vi "ArmController.vi"(7 "Disabled":bool, 9 "Robot Mode":T1, 10 "SensorInputData":T6, 11 "HMI to Control":T2={"RightDriveValue"=0.0, "LeftDriveValue"=0.0, "Arm Manual "=0.0, "Stacker Manual "=0.0, "Claw Manual "=0.0, "ClawSlightOpenNumber"=0, "Intake Value "=0.0, "Arm States"=enum."4 Tote", "Claw States"=enum."Claw Manual ", "Intake Man. or Sense"=enum."Sensing", "Stacker in Manual?"=FALSE, "Drop Stack? "=FALSE, "Tusk Up Request"=FALSE, "Tusk Down Request"=FALSE, "Inver. Wheels  In Request"=FALSE, "Inverse. Wheels Out Request "=FALSE, "Get Out of Manual Control"=FALSE, "Exit Score State"=FALSE, "DriveStraight Help?"=FALSE, "Stacker Shut Off No."=0, "Stacker Need Off?"=FALSE, "Collecting?"=FALSE, "Go to Hover"=FALSE, "Stack Clamp Lock "=FALSE, "Stack Clamp Unlock "=FALSE, "Claw Intake Value "=0.0, "Stack Clamp Lock No. "=0, "Steal Can (ruin their day?)"=FALSE, "Retract (have mercy?)"=FALSE, "Can Grab No. "=0, "Wench Value to Control "=0.0}) -> (2 "Device has arrived":bool, 3 "Final Arm Output":dbl)   [LabVIEW 2014]
uses:
  Typedefs/SensorInputData.ctl
  Typedefs/HMI_to_Control.ctl
  Typedefs/Arm States.ctl
  Typedefs/ClawStates.ctl
  Typedefs/IntakeWheelSenseOrManual.ctl
  <vilib>/Rock Robotics/WPI/DriverStation/WPI_DriverStationRobotMode2.ctl
  Gensubs/Bert_or_Ernie.vi
panel:
  in  "Ramp":dbl=0.04
  in  "permissable arm error range":dbl=1.0 format="%#_13g"
  out "Setpoint, Current Angle, Chart":cluster{"ArmAngle":dbl, "Setpoint ":dbl}(graph)
  out "P,I,D, Total Error, Chart":cluster{"P":dbl, "I":dbl, "D":dbl, "P+I+D":dbl}(graph)
  in  "I Deadband":dbl=3.0
  # "Andrew's Notes:\nGain scheduling should be done in here\nPosition indexing could be done in here"
  # "Setpoint"
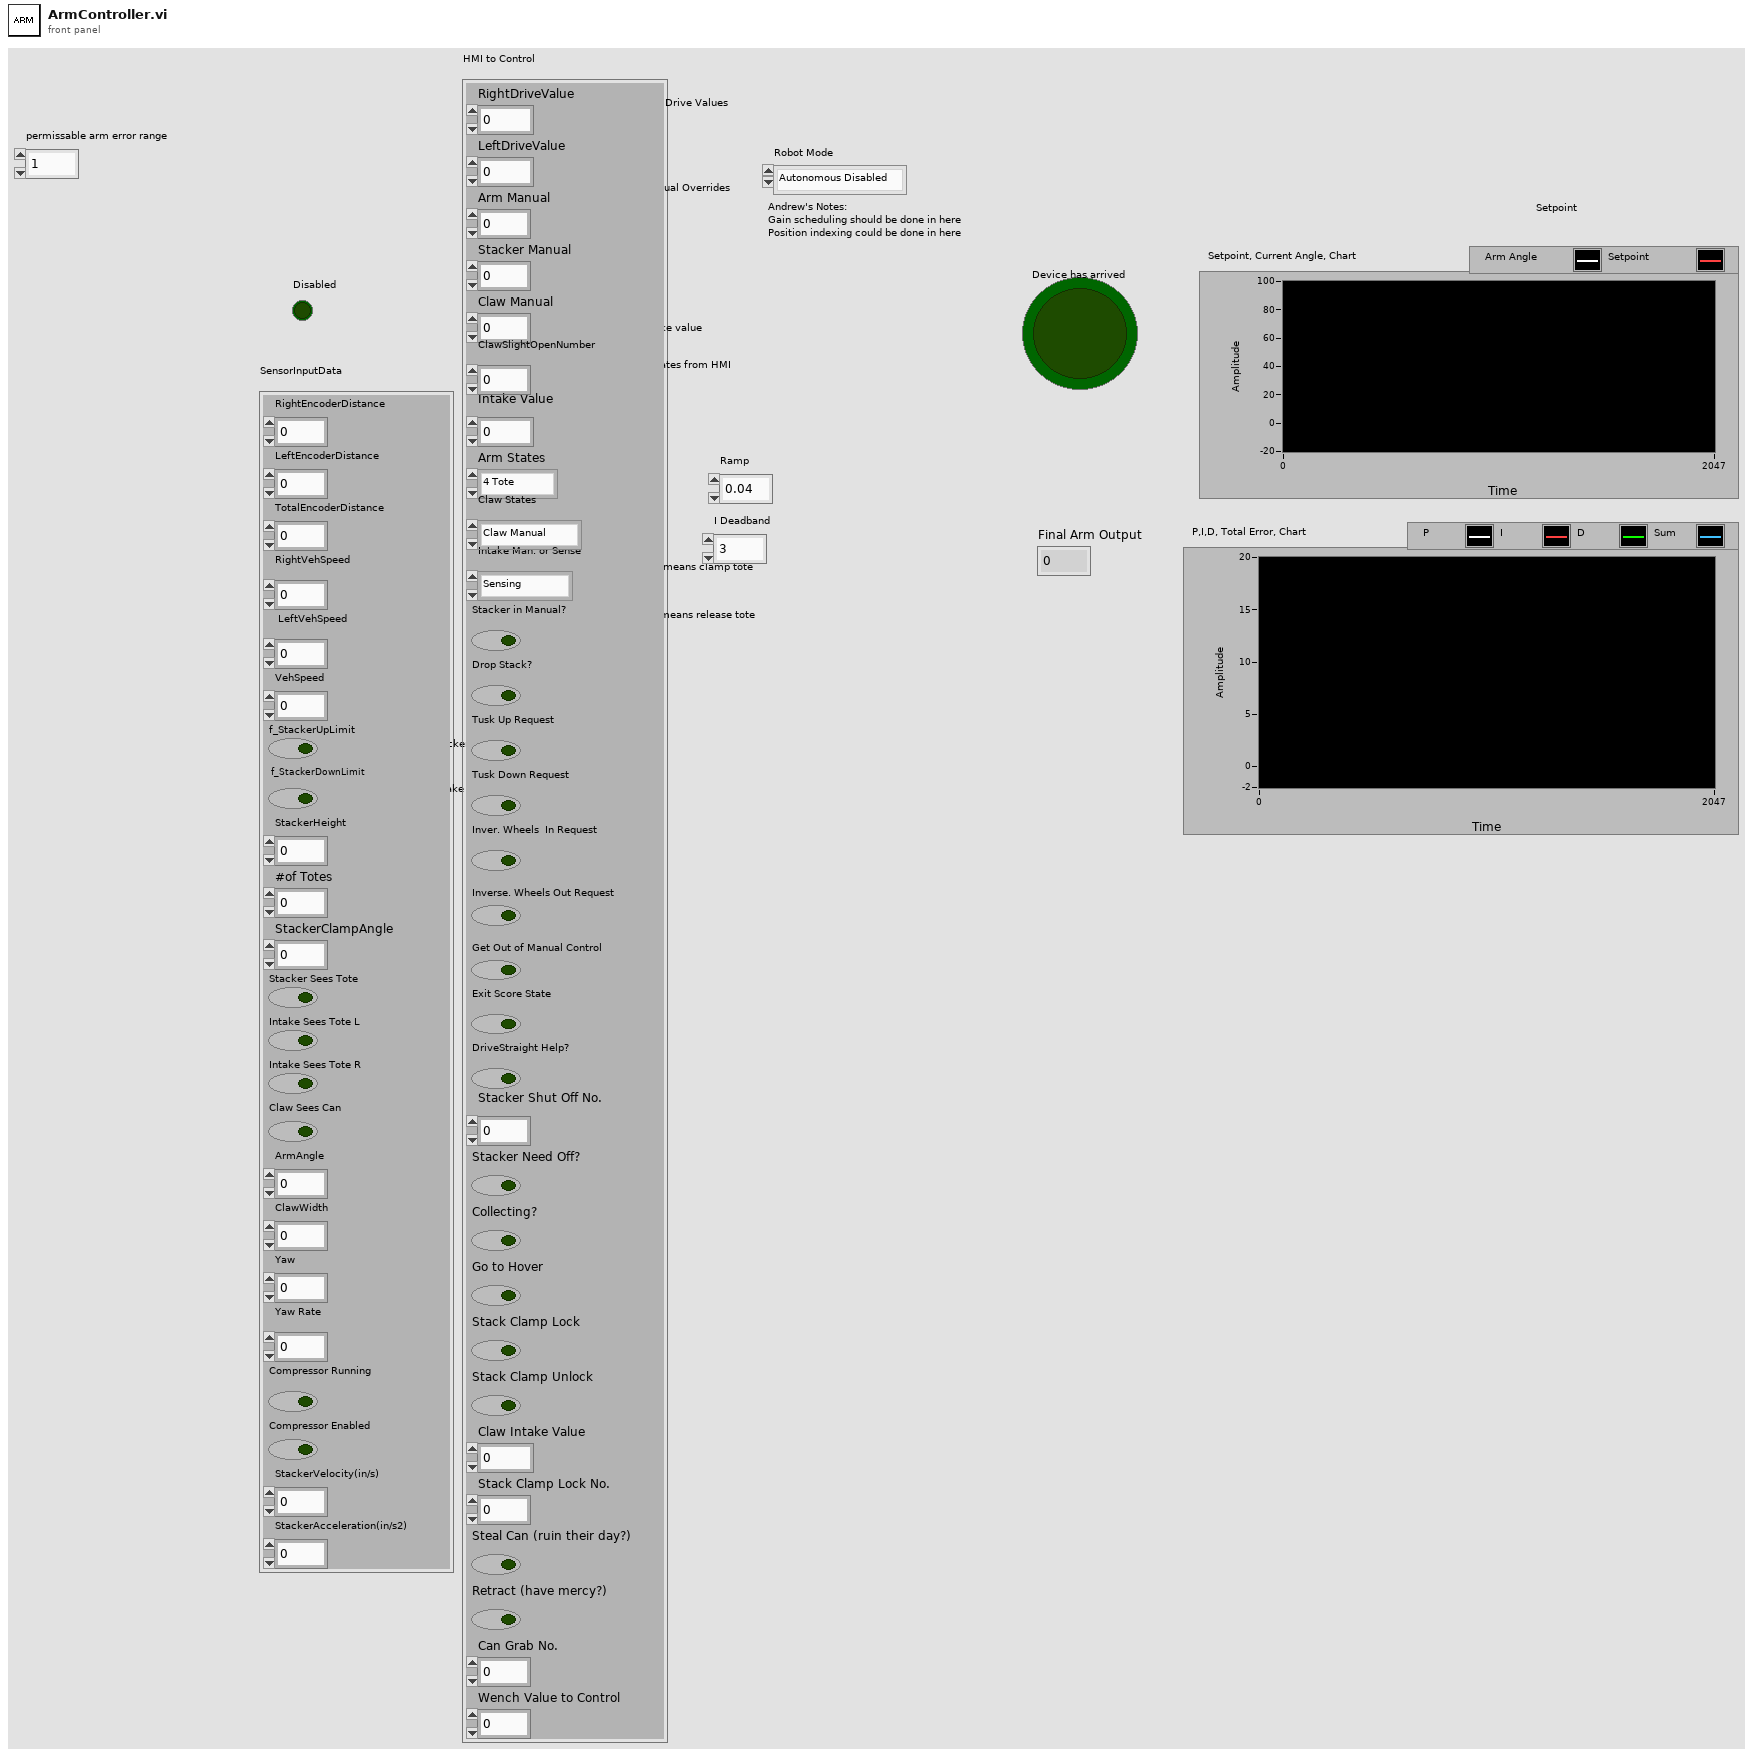
[diagram p1: front panel]
types:
  T1 = typedef "WPI_DriverStationRobotMode2.ctl" = enum16{"Autonomous Disabled", "Autonomous Enabled", "Teleop Disabled", "Teleop Enabled", "Disconnected", "Finish", "Test Disabled", "Test Enabled", "Emergency Stopped"}
  T2 = typedef "HMI_to_Control.ctl" = cluster{"RightDriveValue":dbl, "LeftDriveValue":dbl, "Arm Manual ":dbl, "Stacker Manual ":dbl, "Claw Manual ":dbl, "ClawSlightOpenNumber":i8, "Intake Value ":sgl, "Arm States":T3, "Claw States":T4, "Intake Man. or Sense":T5, "Stacker in Manual?":bool, "Drop Stack? ":bool, "Tusk Up Request":bool, "Tusk Down Request":bool, "Inver. Wheels  In Request":bool, "Inverse. Wheels Out Request ":bool, "Get Out of Manual Control":bool, "Exit Score State":bool, "DriveStraight Help?":bool, "Stacker Shut Off No.":i8, "Stacker Need Off?":bool, "Collecting?":bool, "Go to Hover":bool, "Stack Clamp Lock ":bool, "Stack Clamp Unlock ":bool, "Claw Intake Value ":sgl, "Stack Clamp Lock No. ":i8, "Steal Can (ruin their day?)":bool, "Retract (have mercy?)":bool, "Can Grab No. ":i8, "Wench Value to Control ":dbl}
  T3 = typedef "Arm States.ctl" = enum16{"Arm Manual ", "Ground", "Step", "1 Tote", "2 Tote", "3 Tote", "4 Tote", "5 Tote", "6 Tote", "Flip Can Arm", "Grab Can in auto", "Nudge"}
  T4 = typedef "ClawStates.ctl" = enum16{"Claw Manual ", "Claw Open", "Claw Closed", "Claw Slight Open", "Flip Can"}
  T5 = typedef "IntakeWheelSenseOrManual.ctl" = enum16{"Sensing", "Manual "}
  T6 = typedef "SensorInputData.ctl" = cluster{"RightEncoderDistance":dbl, "LeftEncoderDistance":dbl, "TotalEncoderDistance":dbl, "RightVehSpeed":dbl, "LeftVehSpeed":dbl, "VehSpeed":dbl, "f_StackerUpLimit":bool, "f_StackerDownLimit":bool, "StackerHeight":dbl, "#of Totes":u8, "StackerClampAngle":dbl, "Stacker Sees Tote":bool, "Intake Sees Tote L":bool, "Intake Sees Tote R":bool, "Claw Sees Can":bool, "ArmAngle":dbl, "ClawWidth":dbl, "Yaw":dbl, "Yaw Rate":dbl, "Compressor Running":bool, "Compressor Enabled":bool, "StackerVelocity(in/s)":dbl, "StackerAcceleration(in/s2)":dbl}
  T7 = cluster{"Arm_kP":dbl, "Arm_kI":dbl, "Arm_kD":dbl, "Cos Theta Kp":dbl}
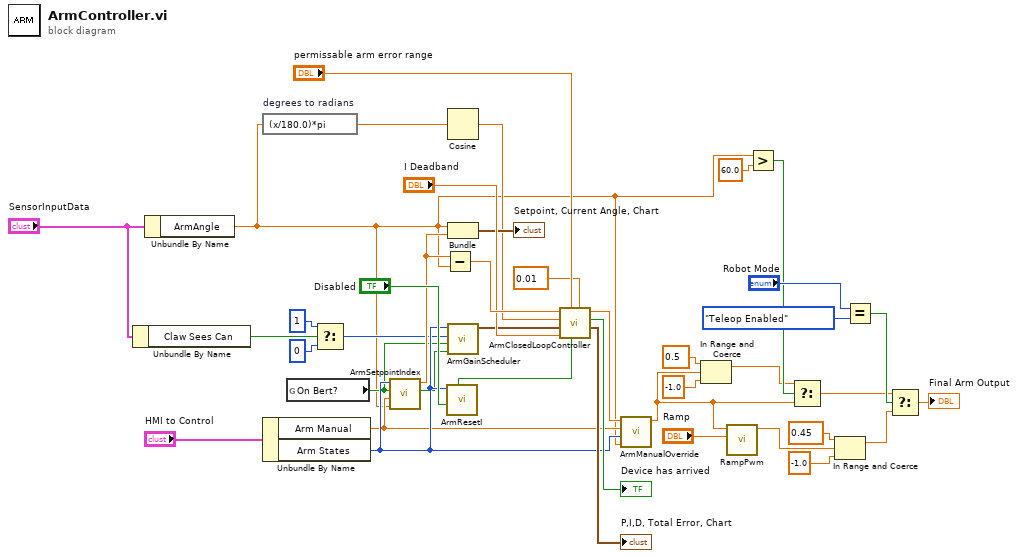
[diagram p0: block diagram]
diagram:
  n1 = Unbundle By Name("SensorInputData") -> ("Claw Sees Can"=w29:bool)
  n2 = Unbundle By Name("SensorInputData") -> ("ArmAngle"=w8:dbl)
  n3 = expression code="(x/180.0)*pi" "degrees to radians"(w8) -> (w23:dbl)
  n4 = Unbundle By Name("HMI to Control") -> ("Arm Manual"=w19:dbl, "Arm States"=w31:T3)
  n5 = global read "Bert_or_Ernie.vi" "On Bert?"() -> (w24:bool)
  n6 = Select(t=1, s=w29, f=0) -> (s? t:f=w26:i32)
  n7 = call "ArmSetpointIndex.vi"("ArmCurrent"=w8, "Joystick Input"=w19, "On Bert?"=w24, "Arm State"=w31) -> ("Lock Setpoint as Current Height"=w18:bool, "Setpoint"=w33:dbl)  [unwired: 6 in]
  n8 = Subtract(x=w33, y=w8) -> (x-y=w36:dbl)
  n9 = call "ArmResetI.vi"("Disabled?"="Disabled", "ArmState"=w31) -> ("Reset I"=w38:bool)  [unwired: 9 in]
  n10 = Cosine(x=w23) -> (cos(x)=w22:dbl)
  n11 = Bundle("ArmAngle"=w8, "Setpoint"=w33) -> (→"Setpoint, Current Angle, Chart":cluster{"ArmAngle":dbl, "Setpoint ":dbl})  [unwired: 1 in]
  n12 = call "ArmGainScheduler.vi"("Lock Setpoint as Current Height"=w18, "On Bert?"=w24, "Have Can?"=w26, "Arm States"=w31) -> ("Arm Gains Out"=w20:T7)  [unwired: 7 in]
  n13 = call "ArmClosedLoopController.vi"("Loop Period"=0.01, "Reset I?"=w38, "permissable error range"="permissable arm error range", "I Deadband"="I Deadband", "Gains"=w20, "Cos of Arm Theta"=w22, "Error"=w36) -> ("PID Variables"=→"P,I,D, Total Error, Chart":cluster{"P":dbl, "I":dbl, "D":dbl, "P+I+D":dbl}, "Device has arrived"=→"Device has arrived":bool, "Output"=w37:dbl)  [unwired: 2 in]
  n14 = call "ArmManualOverride.vi"("ArmAngleIn"=w8, "Arm State"=w31, "Arm Manual"=w19, "Arm Output"=w37) -> ("Final Arm Output"=w2:dbl)  [unwired: 7 in]
  n15 = In Range and Coerce(upper limit=0.5, x=w2, lower limit=-1.0) -> (coerced(x)=w1:dbl)  [unwired: 1 out]
  n16 = call "RampPwm.vi"("Ramp Step"="Ramp", "Input"=w2) -> ("Output"=w14:dbl)  [unwired: 9 in]
  n17 = Greater?(x=w8, y=60.0) -> (0:w6:bool)
  n18 = Select(t=w1, s=w6, f=w2) -> (s? t:f=w5:dbl)
  n19 = In Range and Coerce(upper limit=0.45, x=w14, lower limit=-1.0) -> (coerced(x)=w9:dbl)  [unwired: 1 out]
  n20 = Equal?(x="Robot Mode", y=WPI_DriverStationRobotMode2."Teleop Enabled" ("Robot Mode 2")) -> (x = y?=w10:bool)
  n21 = Select(t=w5, s=w10, f=w9) -> (s? t:f=→"Final Arm Output":dbl)
